vi "Multiple Occurence.vi"() -> ()   [LabVIEW 2010]
panel:
  out "Numeric 3":i32
  out "Numeric 2":i32
  out "Numeric":i32
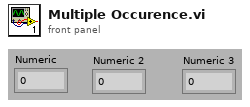
[diagram p1: front panel]
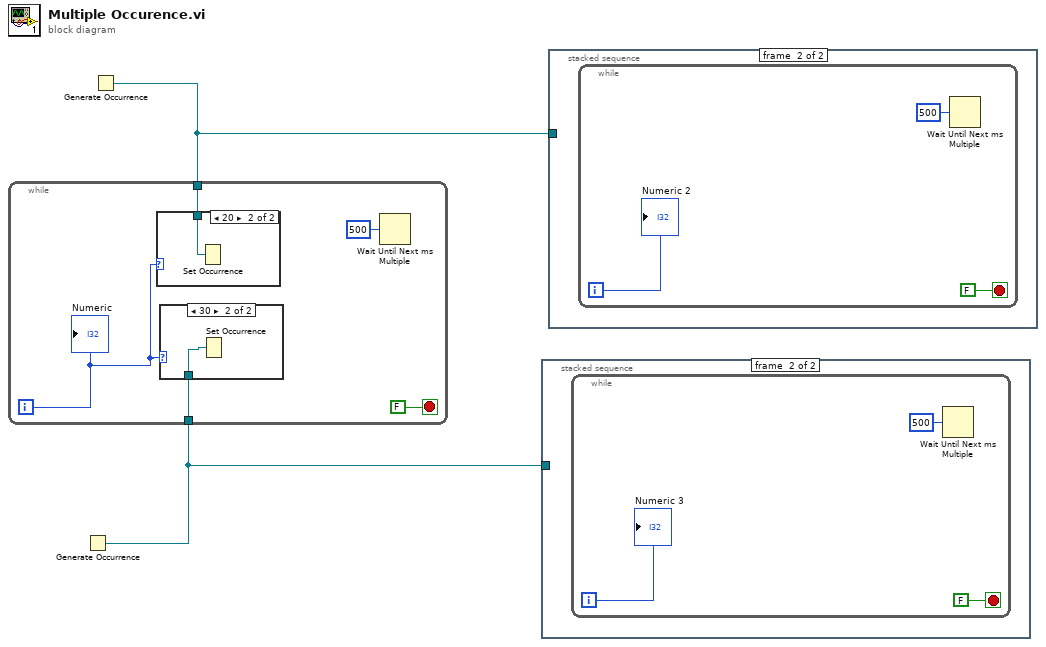
[diagram p0: block diagram]
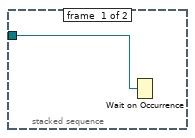
[diagram p2: hidden frame]
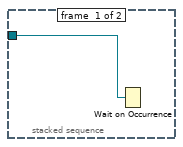
[diagram p3: hidden frame]
diagram:
  n1 = Generate Occurrence() -> (w1:refnum<k4>)
  n2 = Generate Occurrence() -> (w2:refnum<k4>)
  n3 = while {
    tunnel: w2 -> [w4]
    tunnel: w1 -> [w3]
    i -> [w5]
    stop <- FALSE stop-if-true
    n4 = case shown="20" w5 {
      tunnel: w4 -> [_ w9]
      frame 0, Default {
      }
      frame 20 {
        n5 = Set Occurrence(w9) -> ()
      }
    }
    n6 = case shown="30" w5 {
      tunnel: w3 -> [_ w8]
      frame 0, Default {
      }
      frame 30 {
        n7 = Set Occurrence(w8) -> ()
      }
    }
    n8 = Wait Until Next ms Multiple(millisecond multiple=u32 500) -> ()  [unwired: 1 out]
    "Numeric" <- w5
  }
  n9 = stacked-sequence {
    tunnel: w1 -> [w10 _]
    frame #0 {
      n10 = Wait on Occurrence(2:w10) -> ()  [unwired: 2 in, 1 out]
    }
    frame #1 {
      n11 = while {
        i -> [w12]
        stop <- FALSE stop-if-true
        n12 = Wait Until Next ms Multiple(millisecond multiple=u32 500) -> ()  [unwired: 1 out]
        "Numeric 3" <- w12
      }
    }
  }
  n13 = stacked-sequence {
    tunnel: w2 -> [w14 _]
    frame #0 {
      n14 = Wait on Occurrence(2:w14) -> ()  [unwired: 2 in, 1 out]
    }
    frame #1 {
      n15 = while {
        i -> [w16]
        stop <- FALSE stop-if-true
        n16 = Wait Until Next ms Multiple(millisecond multiple=u32 500) -> ()  [unwired: 1 out]
        "Numeric 2" <- w16
      }
    }
  }
